vi "Authentication Schemes.vi"(8 "Error In":errorcluster, 10 "Username":string, 11 "Session In":refnum<class "Session.lvclass">) -> (0 "Error Out":errorcluster, 2 "Supported Schemes":T1[](array[typedef]), 3 "Sesssion Out":refnum<class "Session.lvclass">)   [LabVIEW 2021, in "Field_RnD_Services_LIBSSH2_Toolkit.lvlib" / "Session.lvclass"]
doc: "Gets a list of authentication methods supported by the remote SSH server for a user."
uses:
  Session.lvclass
  Field_RnD_Services_LIBSSH2_Toolkit.lvlib
  SSH/SSH.lvclass
  Type Definitions/User Authentication Schemes.ctl
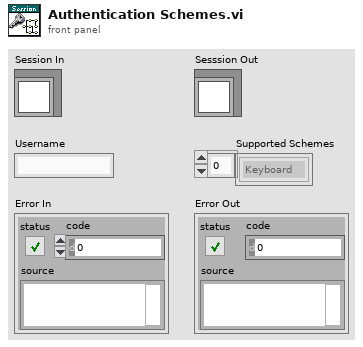
[diagram p1: front panel]
types:
  T1 = typedef "Field_RnD_Services_LIBSSH2_Toolkit.lvlib/Session.lvclass/User Authentication Schemes.ctl" = enum16{"Keyboard", "Password", "Public Key"}
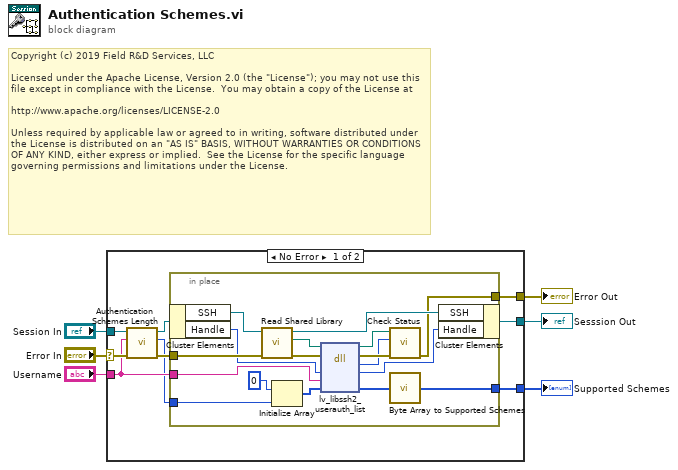
[diagram p0: block diagram]
diagram:
  # "Copyright (c) 2019 Field R&D Services, LLC\n\nLicensed under the Apache License, Version 2.0 (the \"License\"); you may not use this file except in compliance with the License.  You may obtain a copy of the License at\n\nhttp://www.apache.org/licenses/LICENSE-2.0\n\nUnless required by applicable law or agreed to in writing, software distributed under the License is distributed on an \"AS IS\" BASIS, WITHOUT WARRANTIES OR CONDITIONS OF ANY KIND, either express or implied.  See the License for the specific language governing permissions and limitations under the License."
  n1 = case shown="No Error" "Error In" {
    selector: "Error In" -> [w14 w34]
    tunnel: [w7 w34] -> w5
    tunnel: "Session In" -> [w12 w33]
    tunnel: [w15 w33] -> w3
    tunnel: "Username" -> [w10 _]
    tunnel: [w8 _] -> w1
    frame No Error {
      n2 = call "Authentication Schemes Length.vi"("Error In"=w14, "Username"=w10, "Session In"=w12) -> ("Error Out"=w13:errorcluster, "Length"=w9:i32, "Sesssion Out"=w11:refnum<class "Session.lvclass">)  [unwired: 6 in]
      n3 = in-place {
        in-place-border: w13 -> [w29]
        in-place-border: w10 -> [w28]
        in-place-border: w9 -> [w25]
        in-place-border: [w21] -> w8
        in-place-border: [w16] -> w7
        n4 = in-place-cluster #1(w11) -> ("SSH"=w19:refnum<class "SSH.lvclass">, "Handle"=w27:u64)
        n5 = call "Read Shared Library.vi"("Error In"=w29, "SSH In"=w19) -> ("Error Out"=w20:errorcluster, "libssh2lv Shared Library"=w17:path, "SSH Out"=w18:refnum<class "SSH.lvclass">)  [unwired: 7 in]
        n6 = Initialize Array(u8 0, w25) -> (w23:u8[])
        n7 = dll-call lib="D:/Users/cfield/Code/Field R&D Services/SSH/LV-LIBSSH2/LabVIEW/trunk/src/Toolkit/Support/lv-libssh2.dll" fn="lv_libssh2_userauth_list"(path in=w17, error in=w20, "session"=w27, "username"=w28, "buffer"=w23) -> (path out=w31:path, error out=w32:errorcluster, "result"=w30:i32, "session"=w26:u64, "buffer"=w22:u8[])  [unwired: 2 in]
        n8 = call "Check Status.vi"("Error In"=w32, "Status"=w30, "libssh2lv Shared Library In"=w31) -> ("Error Out"=w16:errorcluster)  [unwired: 7 in, 1 out]
        n9 = call "Byte Array to Supported Schemes.vi"("Buffer"=w22) -> ("Supported Schemes"=w21:T1[])
        n10 = in-place-cluster #1("SSH"=w18, "Handle"=w26) -> (w15:refnum<class "Session.lvclass">)
      }
    }
    frame Error {
    }
  }
  "Sesssion Out" <- w3
  "Error Out" <- w5
  "Supported Schemes" <- w1
